vi "Change DO.vi"(7 "DO":T1=enum."hanbay_pos", 11 "val_in":bool) -> (2 "DO Long Out":u32, 3 "DO Out":bool[](array[boolean]))   [LabVIEW 2016]
uses:
  Global FPGA DO.ctl
  Global DO.vi
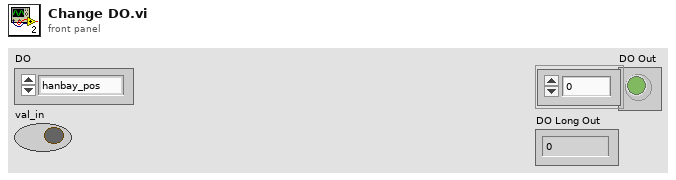
[diagram p1: front panel]
types:
  T1 = typedef "Global FPGA DO.ctl" = enum16{"pas_laser_relay_1", "pas_heater_1", "pas_heater_2", "pas_laser_relay_2", "pas_spk_enable_1", "pas_spk_enable_2", "hanbay_pos", "fan_enable", "crd_laser_enable", "crd_heater_enable", "vacuum_pump", "ac_spare", "uv_enable", "solenoid_1", "solenoid_2", "spare_dc_relay_1", "usb_hub_relay", "spare_dc_relay_2", "fp_aux_1", "fp_aux_2"}
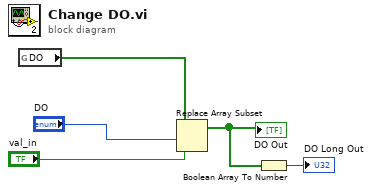
[diagram p0: block diagram]
diagram:
  n1 = global read "Global DO.vi" "DO"() -> (w4:bool[])
  n2 = Replace Array Subset(array=w4, new element="val_in", index="DO") -> (w2:bool[])
  "DO Out" <- w2
  n3 = Boolean Array To Number(Boolean array=w2) -> (number=→"DO Long Out":u32)
